vi "TDMS Reader.vi"() -> ()   [LabVIEW 2010]
panel:
  out "Time of Test":timestamp=timestamp(-9593226000 s since 1904-01-01)
  out "Test Operator":string
  out "Channel Data":waveform(dbl)(graph)
  in  "Data Set":string(combo)="Time Data"
  in  "Serial Number":string
  in  "TDMS File Path":path=path "D:/NI eLearning/LV Core 2/Using TDMS Files/Exercise/Test Data.tdms"
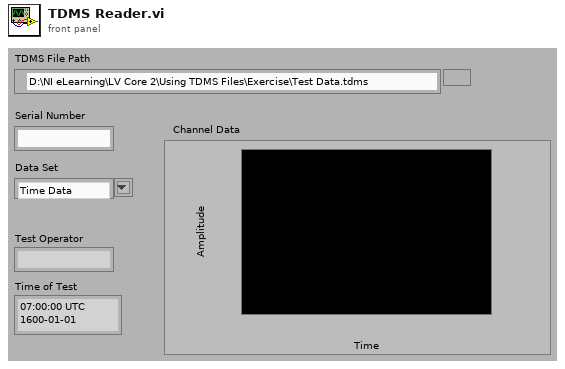
[diagram p1: front panel]
types:
  T1 = enum16{"open", "open or create", "create or replace", "create", "open (read-only)"}
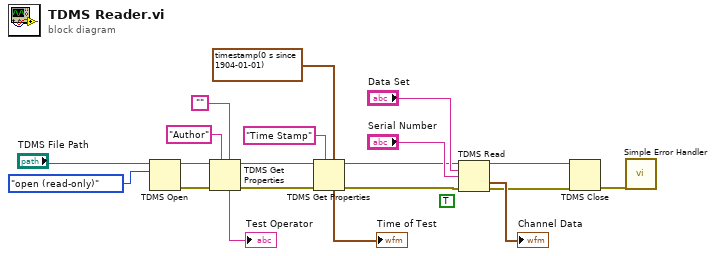
[diagram p0: block diagram]
diagram:
  (unwired) TRUE ("return channels in file order? (F)")
  n1 = TDMS Open(10:T1."open (read-only)" ("operation (0:open)"), 11:"TDMS File Path") -> (0:w12:errorcluster, 3:w13:refnum<k34>)  [unwired: 4 in]
  n2 = TDMS Get Properties(5:"", 7:"Author" ("property name"), 8:w12, 11:w13) -> (0:w9:errorcluster, 3:w11:refnum<k34>, 4:→"Test Operator":string)  [unwired: 5 out]
  n3 = TDMS Get Properties(5:timestamp(0 s since 1904-01-01), 7:"Time Stamp" ("property name"), 8:w9, 11:w11) -> (0:w8:errorcluster, 3:w10:refnum<k34>, 4:→"Time of Test":timestamp)  [unwired: 5 out]
  n4 = TDMS Read(0:w10, 5:"Data Set", 7:"Serial Number", 11:w8) -> (4:w16:refnum<k34>, 10:→"Channel Data":waveform(dbl), 15:w1:errorcluster)  [unwired: 3 in, 3 out]
  n5 = TDMS Close(8:w1, 11:w16) -> (0:w14:errorcluster)  [unwired: 1 out]
  n6 = call <vilib>:"Simple Error Handler.vi"("error in (no error)"=w14) -> ()  [unwired: 1 in, 8 out]
